vi "Log_xml.vi"(0 "ItemName":string, 1 "ItemResult":string, 2 "ItemIndex":i32, 3 "Barcode":string, 4 "BeginDate":string, 5 "EndDate":string, 6 "ParamRes1":string, 7 "Description":string, 8 "ParamRes2":string) -> (16 "Log_xml":string)   [LabVIEW 2014]
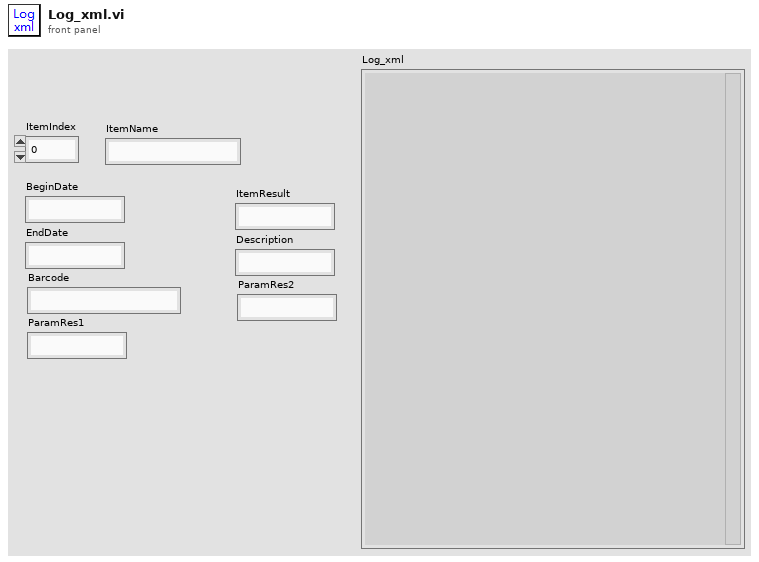
[diagram p1: front panel]
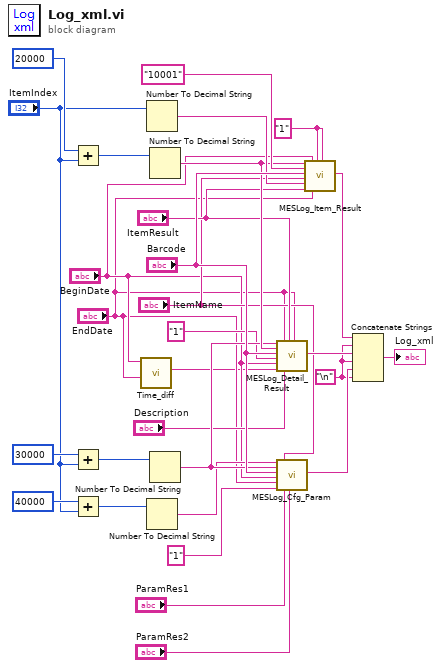
[diagram p0: block diagram]
diagram:
  w1 = "\n"
  w9 = "1" ("ParamResType")
  n1 = Add(x=20000, y="ItemIndex") -> (x+y=w22:i32)
  n2 = Add(x=30000, y="ItemIndex") -> (x+y=w20:i32)
  n3 = Add(x=40000, y="ItemIndex") -> (x+y=w16:i32)
  n4 = call "Time_diff.vi"("End_Time"="EndDate", "Start_Time"="BeginDate") -> ("Time_diff"=w3:string)  [unwired: 9 in]
  n5 = Number To Decimal String(number="ItemIndex") -> (decimal integer string=w24:string)  [unwired: 1 in]
  n6 = Number To Decimal String(number=w16) -> (decimal integer string=w14:string)  [unwired: 1 in]
  n7 = Number To Decimal String(number=w22) -> (decimal integer string=w21:string)  [unwired: 1 in]
  n8 = Number To Decimal String(number=w20) -> (decimal integer string=w18:string)  [unwired: 1 in]
  n9 = call "MESLog_Detail_Result.vi"("DetailResultID"=w18, "ItemResultID"=w21, "Barcode"="Barcode", "LoopID"="1" ("ParamResType"), "BeginDate"="BeginDate", "DiffTime"=w3, "EndDate"="EndDate", "Description"="Description", "DetailResult"="ItemResult", "CreateDate"="EndDate") -> ("Detail_Result"=w28:string)  [unwired: 9 in]
  n10 = call "MESLog_Cfg_Param.vi"("ItemParamID"=w14, "DetailResultID"=w18, "Barcode"="Barcode", "BeginDate"="BeginDate", "EndDate"="EndDate", "ParamResType"="1", "ParamName"="ItemName", "ParamRes1"="ParamRes1", "ParamRes2"="ParamRes2") -> ("Cfg_Param"=w27:string)  [unwired: 10 in]
  n11 = call "MESLog_Item_Result.vi"("ItemResultID"=w21, "ResultID"="10001", "Barcode"="Barcode", "ItemName"="ItemName", "ItemIndex"=w24, "ItemResult"="ItemResult", "BeginDate"="BeginDate", "CreateDate"="EndDate", "LoopNum"=w9, "IsChecked"=w9) -> ("Item_Result"=w29:string)  [unwired: 9 in]
  n12 = Concatenate Strings(w29, w1, w28, w1, w27, w1) -> (→"Log_xml":string)
